vi "Aero_tunnel_monitor_on_OGI.vi"() -> ()   [LabVIEW 2015]
uses:
  Controls/Post_Process.ctl
  <vilib>/Platform/TimedLoop/XDataNode/timing_clust.ctl
  <vilib>/Platform/TimedLoop/XDataNode/nitl_modes.ctl
  <vilib>/Platform/TimedLoop/XDataNode/wakeup.ctl
  ADAM Client/Sub VIs/ADAM Controls/Update_scan_value.ctl
  <vilib>/Utility/file.llb/Write Delimited Spreadsheet (DBL).vi
  Globals/Meas_global.vi
  <vilib>/Platform/TimedLoop/XDataNode/XDataNode.xnode
  <vilib>/Platform/TimedLoop/XDataNode/XDNodeRunTimeDep.lvlib
panel:
  in  "Filename":path
  in  "Duration in Seconds":dbl=30.0
  in  "Log Full Res Balance data":bool
  in  "Use Polynomial for Ratio":bool
  in  "Manual Ratio":dbl=1.0075
  in  "Display Graph?":bool
  in  "Menu Ring":u16(ring) items=["Lift", "Pitch", "Drag", "Side", "Yaw", "Roll"]
  in  "Samples":i32=1000
  out "Waveform Chart":dbl[](graph)
  in  "Output Roll":bool
  out "Roll":string="0.0 Nm"
  in  "Output Yaw":bool
  out "Yaw":string="0.0 Nm"
  in  "Output Pitch":bool
  out "Pitch":string="0.0 Nm"
  in  "Output SF":bool
  out "SF":string="0.0 N"
  in  "Output Drag":bool
  out "Drag":string="0.0 N"
  in  "Output Lift":bool
  out "Lift":string="0.0 N"
  in  "Balance Safety limits":T1(array[cluster])=[{"Max +ve Range"=80, "Max -ve Range"=80, "Axis"="Lift"}, {"Max +ve Range"=80, "Max -ve Range"=80, "Axis"="Pitch"}, {"Max +ve Range"=80, "Max -ve Range"=80, "Axis"="Drag"}, {"Max +ve Range"=80, "Max -ve Range"=80, "Axis"="Side-Force"}, {"Max +ve Range"=99, "Max -ve Range"=99, "Axis"="Yaw"}, {"Max +ve Range"=80, "Max -ve Range"=80, "Axis"="Roll"}] {"Max -ve Range" min=0 max=125; "Max +ve Range" min=0 max=125}
  out "Monitor Speed (Hz)":dbl
  out "Belt slip warning":bool
  out "Road Status":string="???"
  in  "GotoYaw":bool
  in  "NewYawPos":dbl
  out "YAW POSITION":dbl
  out "Required WindSpeedRatio":dbl
  out "ROAD SPEED m/s":dbl
  in  "BL Fan1":i32
  in  "BL Fan2":i32
  in  "Stop drive":bool
  in  "Start Drive":bool
  in  "Synch to Wind":bool
  out "Road Info":string="???"
  in  "stop":bool
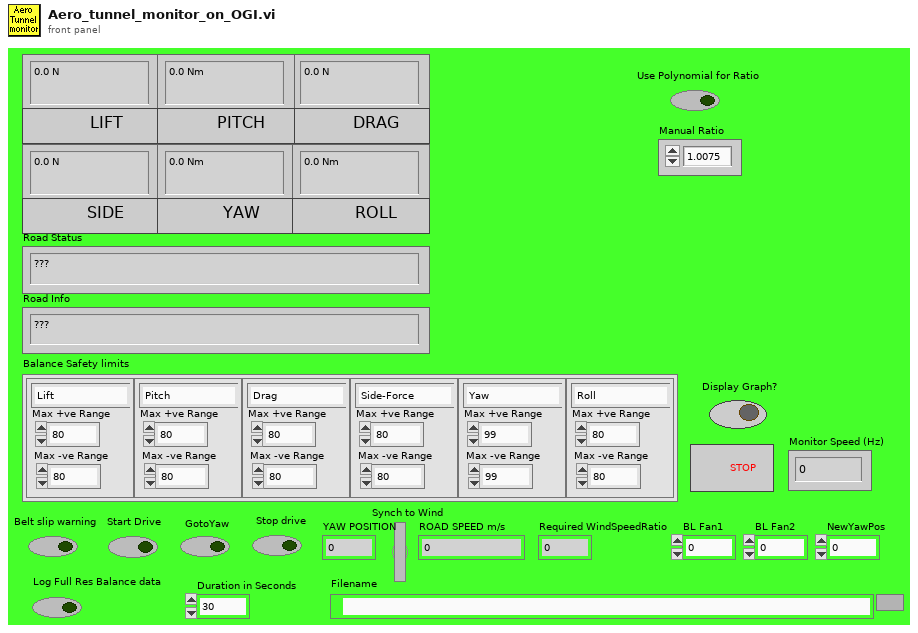
[diagram p1: front panel]
types:
  T1 = cluster{"Max +ve Range":i32, "Max -ve Range":i32, "Axis":string}[]
  T2 = typedef "Post_Process.ctl" = enum16{"Take New Data", "Post Process Raw Data File"}
  T3 = typedef "XDNodeRunTimeDep.lvlib/timing_clust.ctl" = cluster{"Expected End [f-1]":u64, "Actual End [f-1]":u64, "Finished Late? [f-1]":bool, "Expected End [i-1]":u64, "Actual End [i-1]":u64, "Finished Late? [i-1]":bool, "Expected Start [i]":u64, "Actual Start [i]":u64, "Expected Start [f]":u64, "Actual Start [f]":u64, "Source Name":string, "Structure Name":string, "Period":i64, "Deadline":i64, "Offset":i64, "Start":i64, "Priority":i32, "Timeout":i32, "Mode":T4, "Wakeup Reason":T5, "Error":errorcluster, "Source Type":string, "Secondary Source Type":string, "Global End Time":u64, "Global Start Time":u64, "Frame Duration":u64, "Iteration Duration":u64, "Assigned CPU":i32, "I/O Scan Engine Mode":u32}
  T4 = typedef "XDNodeRunTimeDep.lvlib/nitl_modes.ctl" = enum32{"No Change", "Process missed periods, maintain original phase", "Discard missed periods, maintain original phase", "Process missed periods, ignore original phase", "Discard missed periods, ignore original phase"}
  T5 = typedef "XDNodeRunTimeDep.lvlib/wakeup.ctl" = enum32{"Normal", "Aborted", "Asynchronous wakeup", "Timing source error", "Timed loop error", "Timeout"}
  T6 = typedef "Update_scan_value.ctl" = cluster{"Channel Name":string, "New Value":dbl}
  T7 = cluster{"Max +ve Range":i32, "Max -ve Range":i32, "Axis":string}
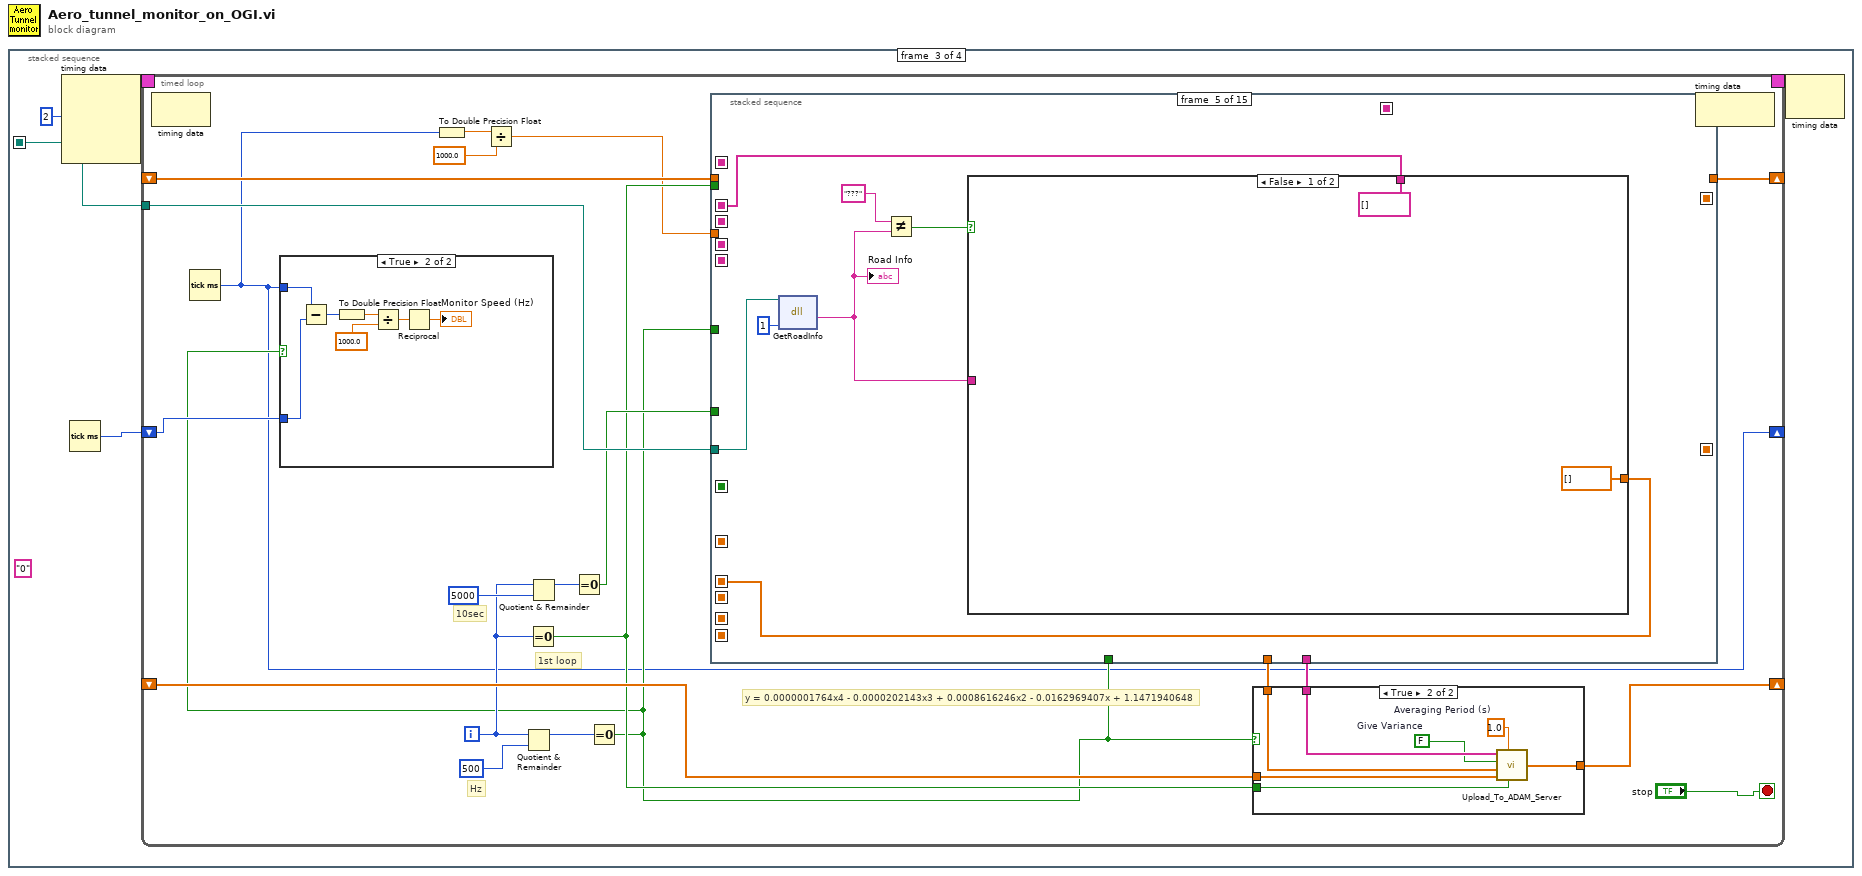
[diagram p0: block diagram]
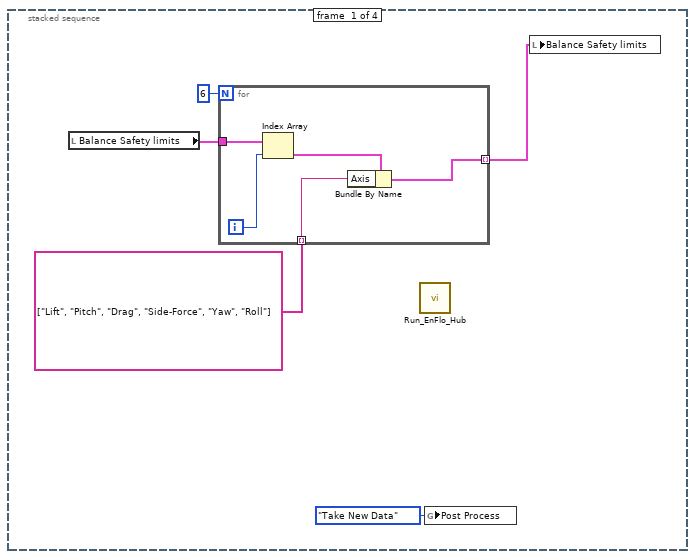
[diagram p2: hidden frame]
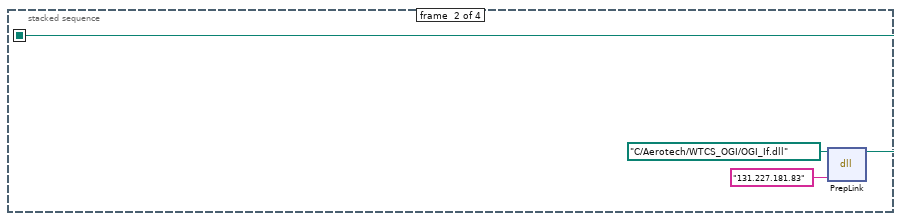
[diagram p3: hidden frame]
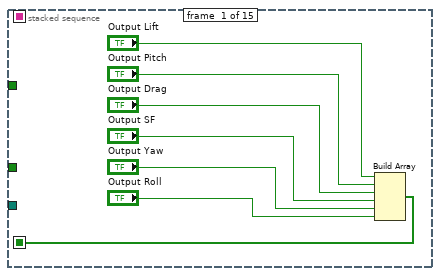
[diagram p6: hidden frame]
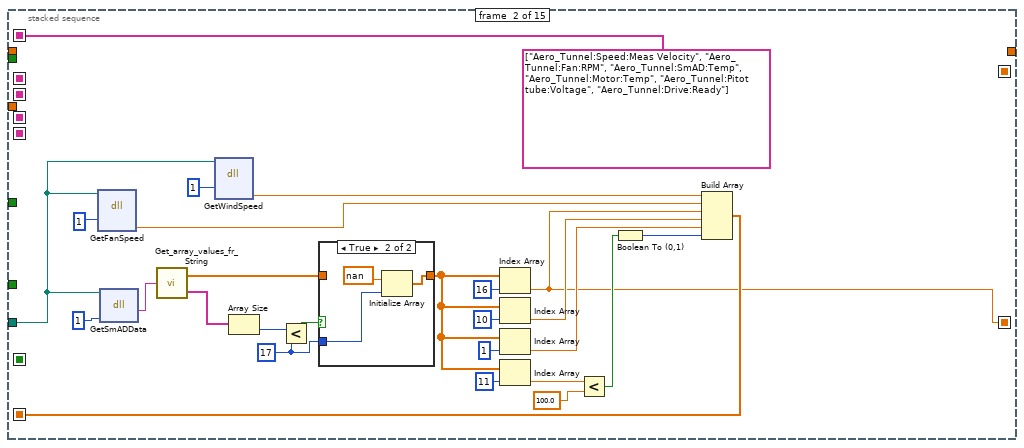
[diagram p7: hidden frame]
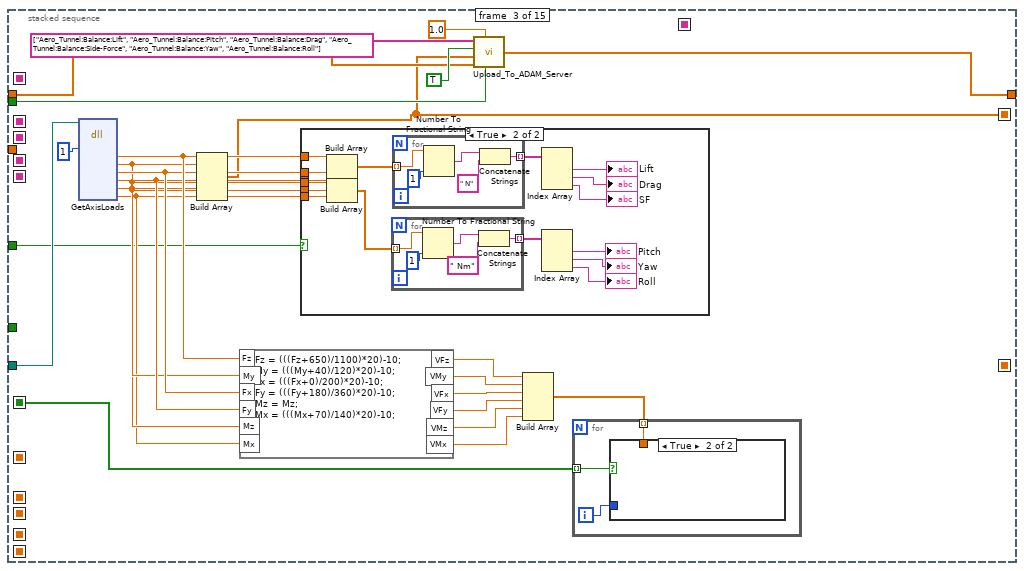
[diagram p9: hidden frame]
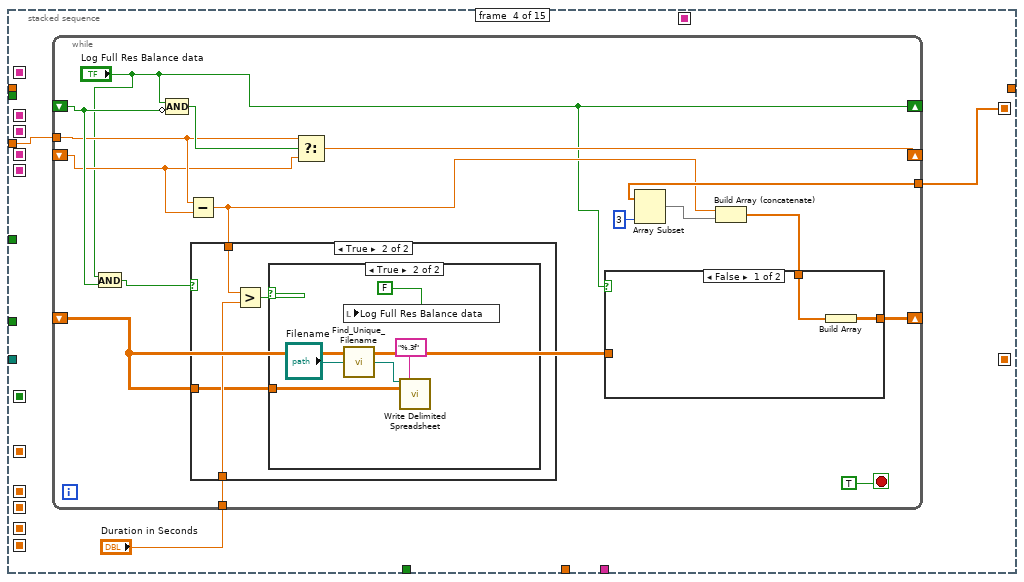
[diagram p12: hidden frame]
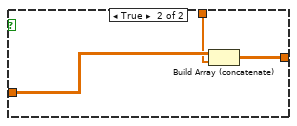
[diagram p13: hidden frame]
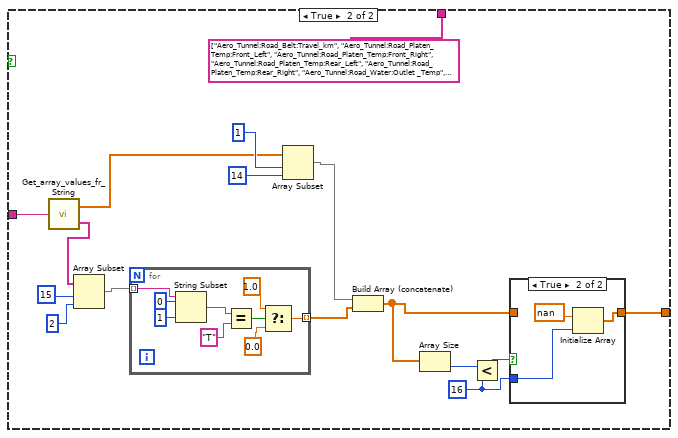
[diagram p16: hidden frame]
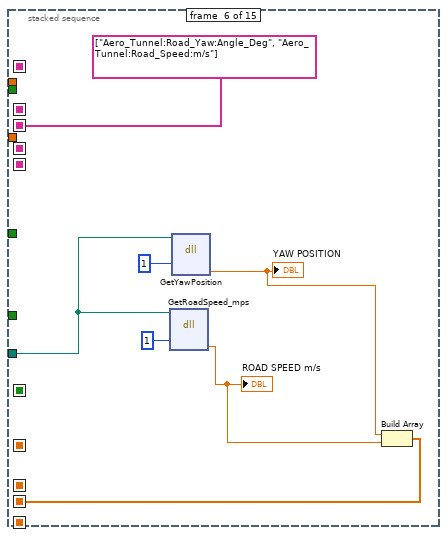
[diagram p18: hidden frame]
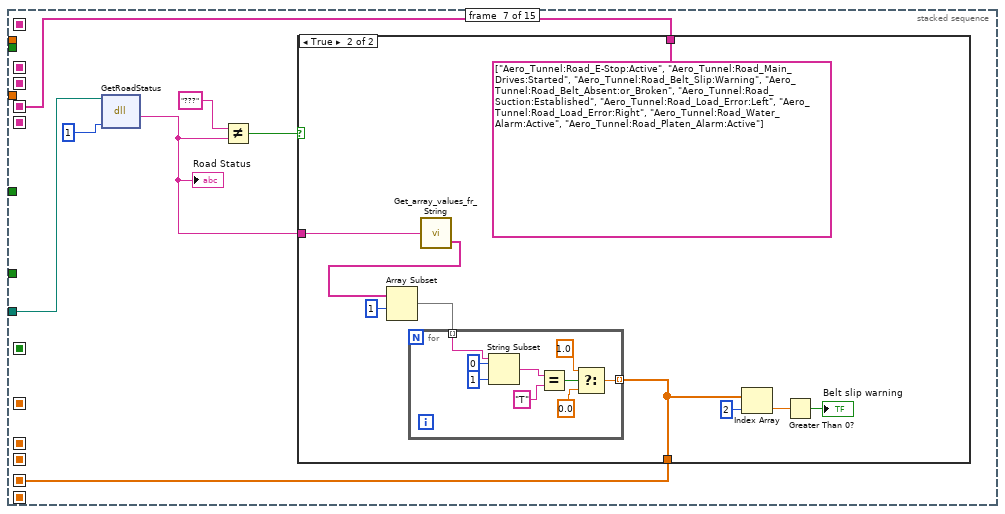
[diagram p19: hidden frame]
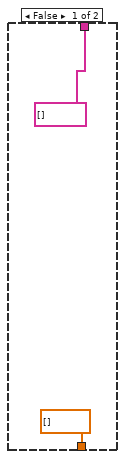
[diagram p20: hidden frame]
diagram:
  n1 = stacked-sequence {
    seq-local: [_ w11 _ _] -> [_ _ w18 w563]
    frame #0 {
      n2 = local read "Balance Safety limits"() -> (w4:T1)
      n3 = for {
        N: 6 -> [_]
        tunnel: w4 -> [w10]
        tunnel: [w7] -> w3 mode=indexing
        tunnel: string[] ["Lift", "Pitch", "Drag", "Side-Force", "Yaw", "Roll"] ("Channel Names") -> [w6] mode=indexing
        i -> [w9]
        n4 = Index Array(array=w10, index=w9) -> (element=w8:T7)
        n5 = Bundle By Name(cluster=w8, "Axis"=w6) -> (w7:T7)
      }
      n6 = call "Run_EnFlo_Hub.vi"() -> ()  [unwired: 8 in]
      n7 = global write "Meas_global.vi" "Post Process"(Post_Process."Take New Data" ("Post Process")) -> ()
      n8 = local write "Balance Safety limits"(w3) -> ()
    }
    frame #1 {
      n9 = dll-call lib="C:/Aerotech/Drivers/OGI_IF.dll" fn="PrepLink"(path in=path "C:/Aerotech/WTCS_OGI/OGI_If.dll", "IPAddress"="131.227.181.83") -> (path out=w11:path)  [unwired: 2 in, 3 out]
    }
    frame #2 {
      (unwired) "0" ("Channels")
      n10 = node-c288(i64 2 ("Period")) -> (w16:T3)  [unwired: 3 in]
      n11 = Tick Count (ms)() -> (millisecond timer value=w17:u32)
      n12 = timed-loop {
        shift-right: [w39] -> _
        shift-left: _ -> [w37]
        tunnel: w18 -> [w35]
        shift-right: [w33] -> _
        shift-left: _ -> [w34]
        timing: w16 -> [_]
        timing-out: [_] -> w15
        shift-right: [w22] -> _
        shift-left: w17 -> [w32]
        i -> [w26]
        stop <- "stop" stop-if-true
        # "1st loop"
        # "10sec"
        # "Hz"
        # "y = 0.0000001764x4 - 0.0000202143x3 + 0.0008616246x2 - 0.0162969407x + 1.1471940648"
        n13 = node-c288() -> ()  [unwired: 1 in, 1 out]
        n14 = Tick Count (ms)() -> (millisecond timer value=w22:u32)
        n15 = To Double Precision Float(number=w22) -> (double precision float=w20:dbl)
        n16 = Divide(x=w20, y=1000.0) -> (x/y=w19:dbl)
        n17 = Quotient & Remainder(x=w26, y=500) -> (x-y*floor(x/y)=w29:i32)  [unwired: 1 out]
        n18 = Equal To 0?(x=w26) -> (x = 0?=w25:bool)
        n19 = Quotient & Remainder(x=w26, y=5000) -> (x-y*floor(x/y)=w28:i32)  [unwired: 1 out]
        n20 = Equal To 0?(x=w28) -> (x = 0?=w27:bool)
        n21 = Equal To 0?(x=w29) -> (x = 0?=w24:bool)
        n22 = case shown="True" w24 {
          tunnel: w32 -> [_ w46]
          tunnel: w22 -> [_ w45]
          frame False {
          }
          frame True {
            n23 = Subtract(x=w45, y=w46) -> (x-y=w44:u32)
            n24 = To Double Precision Float(number=w44) -> (double precision float=w40:dbl)
            n25 = Divide(x=w40, y=1000.0) -> (x/y=w42:dbl)
            n26 = Reciprocal(x=w42) -> (1/x=→"Monitor Speed (Hz)":dbl)
          }
        }
        n27 = stacked-sequence {
          seq-local: [_ string[] ["Aero_Tunnel:Speed:Meas Velocity", "Aero_Tunnel:Fan:RPM", "Aero_Tunnel:SmAD:Temp", "Aero_Tunnel:Motor:Temp", "Aero_Tunnel:Pitot tube:Voltage", "Aero_Tunnel:Drive:Ready"] ("Channel Names") _ _ _ _ _ _ _ _ _ _ _ _ _] -> [_ _ _ _ _ _ _ _ _ _ _ w369 _ _ _]
          seq-local: [_ w79 _ _ _ _ _ _ _ _ _ _ _ _ _] -> [_ _ _ _ _ _ _ _ _ _ _ w368 _ _ _]
          seq-local: [_ _ _ _ w183 _ _ _ _ _ _ _ _ _ _] -> [_ _ _ _ _ _ _ _ _ _ _ w365 _ _ _]
          seq-local: [_ _ _ _ w184 _ _ _ _ _ _ _ _ _ _] -> [_ _ _ _ _ _ _ _ _ _ _ w354 _ _ _]
          seq-local: [_ _ _ _ _ string[] ["Aero_Tunnel:Road_Yaw:Angle_Deg", "Aero_Tunnel:Road_Speed:m/s"] ("Channel Names") _ _ _ _ _ _ _ _ _] -> [_ _ _ _ _ _ _ _ _ _ _ w364 _ _ _]
          seq-local: [_ _ _ _ _ w218 _ _ _ _ _ _ _ _ _] -> [_ _ _ _ _ _ _ _ _ _ _ w363 _ _ _]
          seq-local: [_ _ _ _ _ _ w229 _ _ _ _ _ _ _ _] -> [_ _ _ _ _ _ _ _ _ _ _ w359 _ _ _]
          seq-local: [_ _ _ _ _ _ w228 _ _ _ _ _ _ _ _] -> [_ _ _ _ _ _ _ _ _ _ _ w358 _ _ _]
          seq-local: [w57 _ _ _ _ _ _ _ _ _ _ _ _ _ _] -> [_ _ w109 _ _ _ _ _ _ _ _ _ _ _ _]
          seq-local: [_ _ _ _ _ _ _ string[] ["Aero_Tunnel:Balance_Range:Lift", "Aero_Tunnel:Balance_Range:Pitch", "Aero_Tunnel:Balance_Range:Drag", "Aero_Tunnel:Balance_Range:Side-Force", "Aero_Tunnel:Balance_Range:Yaw", "Aero_Tunnel:Balance_Range:Roll"] ("Channel Names") _ _ _ _ _ _ _] -> [_ _ _ _ _ _ _ _ _ _ _ w355 _ _ _]
          seq-local: [_ _ _ _ _ _ _ w253 _ _ _ _ _ _ _] -> [_ _ _ _ _ _ _ _ w284 _ _ w356 _ _ _]
          seq-local: [_ _ _ _ _ _ _ _ w280 _ _ _ _ _ _] -> [_ _ _ _ _ _ _ _ _ w314 w333 _ _ _ _]
          seq-local: [_ w64 _ _ _ _ _ _ _ _ _ _ _ _ _] -> [_ _ _ _ _ _ _ _ _ _ w332 _ _ _ _]
          seq-local: [_ _ w94 _ _ _ _ _ _ _ _ _ _ _ _] -> [_ _ _ w147 _ _ _ _ _ _ _ _ _ _ _]
          tunnel: [_ _ _ _ _ _ _ _ _ _ _ w367 _ _ _] -> w38
          tunnel: [_ _ _ _ _ _ _ _ _ _ _ w366 _ _ _] -> w36
          tunnel: w35 -> [_ w71 w116 _ w185 w221 w230 w262 _ _ _ w357 w371 w466 w493]
          tunnel: w24 -> [_ _ _ _ _ _ _ _ _ _ _ _ _ _ _]
          tunnel: w34 -> [_ _ w104 _ _ _ _ _ _ _ _ _ _ _ _]
          tunnel: [_ _ w103 _ _ _ _ _ _ _ _ _ _ _ _] -> w33
          tunnel: w24 -> [_ _ w96 _ _ _ _ _ _ _ _ _ w370 _ w492]
          tunnel: w27 -> [_ _ _ _ _ _ _ _ _ w313 _ _ _ w465 _]
          tunnel: w25 -> [_ _ w95 _ _ _ _ _ _ _ _ _ _ _ _]
          tunnel: w19 -> [_ _ _ w149 _ _ _ _ _ _ _ _ _ _ _]
          frame #0 {
            n28 = Build Array("Output Lift", "Output Pitch", "Output Drag", "Output SF", "Output Yaw", "Output Roll") -> (w57:bool[])
          }
          frame #1 {
            w65 = 17 ("y")
            n29 = dll-call lib="C:/Aerotech/Drivers/OGI_IF.dll" fn="GetFanSpeed"(path in=w71, "Enable"=1) -> ("FanSpeedinRPM"=w73:dbl)  [unwired: 3 in, 4 out]
            n30 = dll-call lib="C:/Aerotech/Drivers/OGI_IF.dll" fn="GetSmADData"(path in=w71, "Enable"=1) -> ("SmAD Data String"=w76:string)  [unwired: 2 in, 3 out]
            n31 = call "Get_array_values_fr_String.vi"("String Value"=w76) -> ("Numeric Array"=w66:dbl[], "String array"=w69:string[])
            n32 = dll-call lib="C:/Aerotech/Drivers/OGI_IF.dll" fn="GetWindSpeed"(path in=w71, "Enable"=1) -> ("Windspeed_M/s"=w72:dbl)  [unwired: 3 in, 4 out]
            n33 = Array Size(array=w69) -> (size(s)=w70:i32)
            n34 = Less?(x=w70, y=w65) -> (x < y?=w68:bool)
            n35 = case shown="True" w68 {
              tunnel: [w90 w93] -> w67
              tunnel: w66 -> [w90 _]
              tunnel: w65 -> [_ w91]
              frame False {
              }
              frame True {
                n36 = Initialize Array(nan, w91) -> (w93:dbl[])
              }
            }
            n37 = Index Array(array=w67, index=16) -> (element=w64:dbl)
            n38 = Index Array(array=w67, index=10) -> (element=w87:dbl)
            n39 = Index Array(array=w67, index=1) -> (element=w85:dbl)
            n40 = Index Array(array=w67, index=11) -> (element=w83:dbl)
            n41 = Less?(x=w83, y=100.0) -> (x < y?=w81:bool)
            n42 = Boolean To (0,1)(Boolean=w81) -> (0, 1=w80:i16)
            n43 = Build Array(w72, w73, w64, w87, w85, w80) -> (w79:dbl[])
          }
          frame #2 {
            n44 = dll-call lib="C:/Aerotech/Drivers/OGI_IF.dll" fn="GetAxisLoads"(path in=w116, "Enable"=1) -> ("Lift"=w102:dbl, "Pitch"=w99:dbl, "Drag"=w101:dbl, "side"=w100:dbl, "Yaw"=w98:dbl, "Roll"=w97:dbl)  [unwired: 3 in, 9 out]
            n45 = Build Array(w102, w99, w101, w100, w98, w97) -> (w94:dbl[])
            n46 = formula code="VFz = (((Fz+650)/1100)*20)-10;\nVMy = (((My+40)/120)*20)-10;\nVFx = (((Fx+0)/200)*20)-10;\nVFy = (((Fy+180)/360)*20)-10;\nVMz = Mz;\nVMx = (((Mx+70)/140)*20)-10;"("Fz"=w102, "My"=w99, "Fx"=w101, "Fy"=w100, "Mz"=w98, "Mx"=w97) -> ("VFz"=w115:dbl, "VMy"=w114:dbl, "VFx"=w113:dbl, "VFy"=w112:dbl, "VMz"=w111:dbl, "VMx"=w110:dbl)
            n47 = case shown="True" w96 {
              tunnel: w102 -> [_ w133]
              tunnel: w101 -> [_ w132]
              tunnel: w100 -> [_ w131]
              tunnel: w99 -> [_ w125]
              tunnel: w98 -> [_ w124]
              tunnel: w97 -> [_ w123]
              frame False {
              }
              frame True {
                n48 = Build Array(w133, w132, w131) -> (w130:dbl[])
                n49 = Build Array(w125, w124, w123) -> (w122:dbl[])
                n50 = for {
                  tunnel: w122 -> [w134] mode=indexing
                  tunnel: [w138] -> w121 mode=indexing
                  n51 = Number To Fractional String(number=w134, precision (6)=i16 1) -> (F-format string=w135:string)  [unwired: 2 in]
                  n52 = Concatenate Strings(w135, " Nm" ("string")) -> (w138:string)
                }
                n53 = for {
                  tunnel: w130 -> [w139] mode=indexing
                  tunnel: [w143] -> w129 mode=indexing
                  n54 = Number To Fractional String(number=w139, precision (6)=i16 1) -> (F-format string=w140:string)  [unwired: 2 in]
                  n55 = Concatenate Strings(w140, " N" ("string")) -> (w143:string)
                }
                n56 = Index Array(array=w129) -> (element #1=→"Lift":string, element #2=→"Drag":string, element #3=→"SF":string)  [unwired: 3 in]
                n57 = Index Array(array=w121) -> (element #1=→"Pitch":string, element #2=→"Yaw":string, element #3=→"Roll":string)  [unwired: 3 in]
              }
            }
            n58 = call "Upload_To_ADAM_Server.vi"("First Loop"=w95, "Averaging Period (s)"=1.0, "Shift In"=w104, "Channel Values"=w94, "Give Variance"=TRUE, "Channel Names"=string[] ["Aero_Tunnel:Balance:Lift", "Aero_Tunnel:Balance:Pitch", "Aero_Tunnel:Balance:Drag", "Aero_Tunnel:Balance:Side-Force", "Aero_Tunnel:Balance:Yaw", "Aero_Tunnel:Balance:Roll"]) -> ("Shift Out"=w103:dbl[])
            n59 = Build Array(w115, w114, w113, w112, w111, w110) -> (w108:dbl[])
            n60 = for {
              tunnel: w109 -> [w146] mode=indexing
              tunnel: w108 -> [w145] mode=indexing
              i -> [w144]
              n61 = case shown="True" w146 {
                tunnel: w145 -> [_ _]
                tunnel: w144 -> [_ _]
                frame False {
                }
                frame True {
                }
              }
            }
          }
          frame #3 {
            n62 = while {
              shift-right: ["Log Full Res Balance data"] -> _
              shift-left: _ -> [w163]
              shift-right: [w164] -> _
              shift-left: _ -> [w157]
              tunnel: w149 -> [w158]
              tunnel: "Duration in Seconds" -> [w161]
              tunnel: w147 -> [w159]
              shift-right: [w155] -> _
              shift-left: _ -> [w150]
              stop <- TRUE stop-if-true
              n63 = And(x="Log Full Res Balance data", y=w163) -> (x .and. y?=w162:bool)
              n64 = Compound Arithmetic op=AND("Log Full Res Balance data", invert w163) -> (w165:bool)
              n65 = Subtract(x=w158, y=w157) -> (x-y=w156:dbl)
              n66 = case shown="True" w162 {
                tunnel: w161 -> [_ w174]
                tunnel: w156 -> [_ w172]
                tunnel: w150 -> [_ w171]
                frame False {
                }
                frame True {
                  n67 = Greater?(x=w172, y=w174) -> (0:w173:bool)
                  n68 = case shown="True" w173 {
                    tunnel: w171 -> [_ w178]
                    frame False {
                    }
                    frame True {
                      n69 = local write "Log Full Res Balance data"(FALSE) -> ()
                      n70 = call "Find_Unique_Filename.vi"("Path In"="Filename") -> ("Unique Path Out"=w176:path)  [unwired: 2 in]
                      n71 = call-poly <vilib>:"Write Delimited Spreadsheet.vi"("file path (dialog if empty)"=w176, "format (%.3f)"="%.3f", "2D data"=w178) -> ()  [unwired: 11 in, 2 out]
                    }
                  }
                }
              }
              n72 = Select(t=w158, s=w165, f=w157) -> (s? t:f=w164:dbl)
              n73 = Array Subset(array=w159, length=3) -> (w153:dbl[])  [unwired: 1 in]
              n74 = Build Array (concatenate)(w156, w153) -> (w152:dbl[])
              n75 = case shown="False" "Log Full Res Balance data" {
                tunnel: [w166 w170] -> w155
                tunnel: w150 -> [_ w169]
                tunnel: w152 -> [w167 w168]
                frame False {
                  n76 = Build Array(w167) -> (w166:dbl[][])
                }
                frame True {
                  n77 = Build Array (concatenate)(w169, w168) -> (w170:dbl[][])
                }
              }
            }
          }
          frame #4 {
            n78 = dll-call lib="C:/Aerotech/Drivers/OGI_IF.dll" fn="GetRoadInfo"(path in=w185, "Enable"=1) -> ("Road Info"=w181:string)  [unwired: 3 in, 2 out]
            "Road Info" <- w181
            n79 = Not Equal?(x="???", y=w181) -> (x != y?=w180:bool)
            n80 = case shown="False" w180 {
              tunnel: [string[] [] ("Channel Names") string[] ["Aero_Tunnel:Road_Belt:Travel_km", "Aero_Tunnel:Road_Platen_Temp:Front_Left", "Aero_Tunnel:Road_Platen_Temp:Front_Right", "Aero_Tunnel:Road_Platen_Temp:Rear_Left", "Aero_Tunnel:Road_Platen_Temp:Rear_Right", "Aero_Tunnel:Road_Water:Outlet _Temp", "Aero_Tunnel:Road_Water:Inlet _Temp", "Aero_Tunnel:Road_Suction:Front", "Aero_Tunnel:Road_Suction:Middle", "Aero_Tunnel:Road_Suction:Rear", "Aero_Tunnel:Road_BL_Suction:Primary", "Aero_Tunnel:Road_BL_Suction:Secondary", "Aero_Tunnel:Road_LoadCell:Left", "Aero_Tunnel:Road_LoadCell:Right", "Aero_Tunnel:Road_Water_High:Temp_Alarm", "Aero_Tunnel:Road_Platen_High:Temp_Alarm"] ("Channel Names")] -> w184
              tunnel: [dbl[] [] w190] -> w183
              tunnel: w181 -> [_ w189]
              frame False {
              }
              frame True {
                w193 = 16 ("y")
                n81 = call "Get_array_values_fr_String.vi"("String Value"=w189) -> ("Numeric Array"=w192:dbl[], "String array"=w196:string[])
                n82 = Array Subset(array=w196, index=15, length=2) -> (w200:string[])
                n83 = for {
                  tunnel: w200 -> [w215] mode=indexing
                  tunnel: [w209] -> w199 mode=indexing
                  n84 = String Subset(string=w215, offset (0)=0, length (rest)=1 ("length (rest)")) -> (substring=w214:string)
                  n85 = Equal?(x=w214, y="T") -> (x = y?=w212:bool)
                  n86 = Select(t=1.0, s=w212, f=0.0) -> (s? t:f=w209:dbl)
                }
                n87 = Array Subset(array=w192, index=1, length=14) -> (w198:dbl[])
                n88 = Build Array (concatenate)(w198, w199) -> (w191:dbl[])
                n89 = Array Size(array=w191) -> (size(s)=w195:i32)
                n90 = Less?(x=w195, y=w193) -> (x < y?=w194:bool)
                n91 = case shown="True" w194 {
                  tunnel: [w205 w208] -> w190
                  tunnel: w191 -> [w205 _]
                  tunnel: w193 -> [_ w206]
                  frame False {
                  }
                  frame True {
                    n92 = Initialize Array(nan, w206) -> (w208:dbl[])
                  }
                }
              }
            }
          }
          frame #5 {
            n93 = dll-call lib="C:/Aerotech/Drivers/OGI_IF.dll" fn="GetRoadSpeed_mps"(path in=w221, "Enable"=1) -> ("RoadSpeed_mps"=w219:dbl)  [unwired: 3 in, 4 out]
            "ROAD SPEED m/s" <- w219
            n94 = dll-call lib="C:/Aerotech/Drivers/OGI_IF.dll" fn="GetYawPosition"(path in=w221, "Enable"=1) -> ("Yaw Position"=w220:dbl)  [unwired: 3 in, 4 out]
            "YAW POSITION" <- w220
            n95 = Build Array(w220, w219) -> (w218:dbl[])
          }
          frame #6 {
            n96 = dll-call lib="C:/Aerotech/Drivers/OGI_IF.dll" fn="GetRoadStatus"(path in=w230, "Enable"=1) -> ("Road Status"=w227:string)  [unwired: 3 in, 2 out]
            "Road Status" <- w227
            n97 = Not Equal?(x="???", y=w227) -> (x != y?=w225:bool)
            n98 = case shown="True" w225 {
              tunnel: [string[] [] ("Channel Names") string[] ["Aero_Tunnel:Road_E-Stop:Active", "Aero_Tunnel:Road_Main_Drives:Started", "Aero_Tunnel:Road_Belt_Slip:Warning", "Aero_Tunnel:Road_Belt_Absent:or_Broken", "Aero_Tunnel:Road_Suction:Established", "Aero_Tunnel:Road_Load_Error:Left", "Aero_Tunnel:Road_Load_Error:Right", "Aero_Tunnel:Road_Water_Alarm:Active", "Aero_Tunnel:Road_Platen_Alarm:Active"] ("Channel Names")] -> w229
              tunnel: [dbl[] [] w241] -> w228
              tunnel: w227 -> [_ w234]
              frame False {
              }
              frame True {
                n99 = call "Get_array_values_fr_String.vi"("String Value"=w234) -> ("String array"=w237:string[])  [unwired: 1 out]
                n100 = Array Subset(array=w237, index=1) -> (w235:string[])  [unwired: 1 in]
                n101 = for {
                  tunnel: [w244] -> w241 mode=indexing
                  tunnel: w235 -> [w243] mode=indexing
                  n102 = String Subset(string=w243, offset (0)=0, length (rest)=1 ("length (rest)")) -> (substring=w249:string)
                  n103 = Equal?(x=w249, y="T") -> (x = y?=w247:bool)
                  n104 = Select(t=1.0, s=w247, f=0.0) -> (s? t:f=w244:dbl)
                }
                n105 = Index Array(array=w241, index=2) -> (element=w239:dbl)
                n106 = Greater Than 0?(x=w239) -> (x > 0?=→"Belt slip warning":bool)
              }
            }
          }
          frame #7 {
            n107 = dll-call lib="C:/Aerotech/Drivers/OGI_IF.dll" fn="GetAxisPercs"(path in=w262, "Enable"=1) -> ("Lift"=w260:dbl, "Pitch"=w259:dbl, "Drag"=w258:dbl, "side"=w257:dbl, "Yaw"=w256:dbl, "Roll"=w255:dbl)  [unwired: 3 in, 9 out]
            n108 = Build Array(w260, w259, w258, w257, w256, w255) -> (w253:dbl[])
            n109 = case shown="True" "Display Graph?" {
              selector: "Display Graph?" -> [w263 w264]
              tunnel: w253 -> [_ w268]
              frame False {
                n110 = property on="Waveform Chart" class="WFChart (strict)"("Visible"=w263) -> ()  [unwired: 2 in, 2 out]
                n111 = property on="Samples" class="DigNum (strict)"("Visible"=w263) -> ()  [unwired: 2 in, 2 out]
                n112 = property on="Menu Ring" class="Ring (strict)"("Visible"=w263) -> ()  [unwired: 2 in, 2 out]
              }
              frame True {
                n113 = while {
                  shift-right: [w270] -> _
                  shift-left: _ -> [w272]
                  tunnel: w268 -> [w271]
                  tunnel: [w270] -> w267
                  stop <- TRUE stop-if-true
                  n114 = for {
                    tunnel: w272 -> [w275]
                    tunnel: w271 -> [w273] mode=indexing
                    tunnel: [w278] -> w270 mode=indexing
                    i -> [w276]
                    n115 = Index Array(array=w275, index (row)=w276) -> (element=w274:dbl[])  [unwired: 1 in]
                    n116 = Build Array (concatenate)(w273, w274) -> (w279:dbl[])
                    n117 = Array Subset(array=w279, length="Samples") -> (w278:dbl[])  [unwired: 1 in]
                  }
                }
                n118 = Index Array(array=w267, index (row)="Menu Ring") -> (element=→"Waveform Chart":dbl[])  [unwired: 1 in]
                n119 = property on="Waveform Chart" class="WFChart (strict)"("Visible"=w264) -> ()  [unwired: 2 in, 2 out]
                n120 = property on="Samples" class="DigNum (strict)"("Visible"=w264) -> ()  [unwired: 2 in, 2 out]
                n121 = property on="Menu Ring" class="Ring (strict)"("Visible"=w264) -> ()  [unwired: 2 in, 2 out]
              }
            }
          }
          frame #8 {
            n122 = for {
              tunnel: "Balance Safety limits" -> [w300] mode=indexing
              tunnel: w284 -> [w303] mode=indexing
              shift-right: [w297] -> w281
              shift-left: "" -> [w298]
              n123 = To Long Integer(number=w303) -> (32bit integer=w299:i32)
              n124 = Unbundle By Name(w300) -> ("Max +ve Range"=w305:i32, "Max -ve Range"=w304:i32)
              n125 = Negate(x=w304) -> (-x=w302:i32)
              n126 = In Range and Coerce(upper limit=w305, x=w299, lower limit=w302) -> (In Range?=w301:bool)  [unwired: 1 out]
              n127 = case shown="False" w301 {
                tunnel: w300 -> [w311 _]
                tunnel: w299 -> [w309 _]
                tunnel: w298 -> [w307 w312]
                tunnel: [w306 w312] -> w297
                frame False {
                  n128 = Unbundle By Name(w311) -> ("Axis"=w310:string)
                  n129 = Format Into String(format string="The %s is at %d%% of its range.\n", initial string=w307, w310, w309) -> (resulting string=w306:string)  [unwired: 1 in, 1 out]
                }
                frame True {
                }
              }
            }
            n130 = Empty String/Path?(string/path=w281) -> (empty?=w282:bool)
            n131 = case shown="False" w282 {
              tunnel: w281 -> [w288 w296]
              tunnel: [w286 w296] -> w280
              frame False {
                n132 = Build Array("Aero_Tunnel:Fan:Watchdog") -> (w295:string[])
                n133 = call "Get_Current_Scan_client.vi"("ADAM Ch Names"=w295) -> ("Numerical Values"=w293:dbl[])  [unwired: 1 in, 2 out]
                n134 = Index Array(array=w293, index=0) -> (element=w291:dbl)
                n135 = Greater?(x=w291, y=0.5) -> (0:w289:bool)
                n136 = Select(t=w288, s=w289, f="") -> (s? t:f=w286:string)
              }
              frame True {
              }
            }
          }
          frame #9 {
            n137 = while {
              tunnel: w314 -> [w318]
              tunnel: w313 -> [w315]
              stop <- TRUE stop-if-true
              n138 = Empty String/Path?(string/path=w318) -> (empty?=w320:bool)
              n139 = Not(x=w320) -> (.not. x?=w316:bool)
              n140 = Compound Arithmetic op=AND(w316, w315) -> (w319:bool)
              n141 = case shown="True" w319 {
                tunnel: w318 -> [_ w325]
                frame False {
                }
                frame True {
                  w324 = string[] ["Aero_Tunnel:Fan:Watchdog", "Aero_Tunnel:Road:Watchdog", "Aero_Tunnel:Speed:Dem Velocity"] ("Channel Names")
                  n142 = Format Into String(format string="The Aero Tunnel balance has gone outside of its limits.\n%s\nThe Aero_Tunnel:Fan:Watchdog has therefore been disabled. ", w325) -> (resulting string=w326:string)  [unwired: 2 in, 1 out]
                  n143 = Bundle By Name(cluster=errorcluster {"status"=TRUE, "code"=0, "source"=""} ("error in (no error)"), "source"=w326) -> (w328:errorcluster)
                  n144 = Array Size(array=w324) -> (size(s)=w323:i32)
                  n145 = call "EnFlo_Error_Handler.vi"("error in (no error)"=w328, "Error Type"="Aero Tunnel Balance Range Trip", "Dialog Box (T)"=FALSE) -> ()  [unwired: 3 out]
                  n146 = Initialize Array(0.0, w323) -> (w321:dbl[])
                  n147 = call "ASYNC_Adam_client.vi"("Values"=w321, "Channel Names"=w324) -> ()  [unwired: 1 in, 2 out]
                }
              }
            }
          }
          frame #10 {
            n148 = while {
              tunnel: w333 -> [_]
              shift-right: [w338] -> _
              shift-left: _ -> [w337]
              tunnel: w332 -> [w335]
              stop <- TRUE stop-if-true
              n149 = Greater?(x=w335, y=35.0) -> (0:w338:bool)
              n150 = Number To Fractional String(number=w335, precision (6)=i16 2) -> (F-format string=w334:string)  [unwired: 2 in]
              n151 = Compound Arithmetic op=AND(invert w337, w338) -> (w341:bool)
              n152 = case shown="True" w341 {
                tunnel: w334 -> [_ w346]
                frame False {
                }
                frame True {
                  w345 = string[] ["Aero_Tunnel:Fan:Watchdog", "Aero_Tunnel:Road:Watchdog", "Aero_Tunnel:Speed:Dem Velocity"] ("Channel Names")
                  n153 = Format Into String(format string="The Aero Tunnel temperature has gone above it's limits and is:\n%s\nThe Aero_Tunnel:Fan:Watchdog has therefore been disabled. ", w346) -> (resulting string=w347:string)  [unwired: 2 in, 1 out]
                  n154 = Bundle By Name(cluster=errorcluster {"status"=TRUE, "code"=0, "source"=""} ("error in (no error)"), "source"=w347) -> (w349:errorcluster)
                  n155 = Array Size(array=w345) -> (size(s)=w344:i32)
                  n156 = call "EnFlo_Error_Handler.vi"("error in (no error)"=w349, "Error Type"="Aero Tunnel Temperature Trip", "Dialog Box (T)"=FALSE) -> ()  [unwired: 3 out]
                  n157 = Initialize Array(0.0, w344) -> (w342:dbl[])
                  n158 = call "ASYNC_Adam_client.vi"("Values"=w342, "Channel Names"=w345) -> ()  [unwired: 1 in, 2 out]
                }
              }
            }
          }
          frame #11 {
            n159 = Build Array (concatenate)(w368, w365, w363, w358, w356) -> (w367:dbl[])
            n160 = Boolean To (0,1)(Boolean="GotoYaw") -> (0, 1=w362:i16)
            n161 = Build Array (concatenate)(w369, w354, w364, w359, w355) -> (w366:string[])
            n162 = To Long Integer(number=w362) -> (32bit integer=w353:i32)
            n163 = dll-call lib="C:/Aerotech/Drivers/OGI_IF.dll" fn="GotoYawPosition"(path in=w357, "Enable"=w353, "NewYawPos"="NewYawPos") -> ()  [unwired: 3 in, 4 out]
          }
          frame #12 {
            n164 = case shown="True" w370 {
              tunnel: w371 -> [_ w372]
              frame False {
              }
              frame True {
                # "Tweak"
                # "Speed"
                # "Tweak"
                # "Speed"
                n165 = stacked-sequence {
                  seq-local: [_ w386 _ _ _ _] -> [_ _ _ w431 _ _]
                  seq-local: [_ w377 _ _ _ _] -> [_ _ _ w427 _ _]
                  seq-local: [_ w384 _ _ _ _] -> [_ _ _ _ w447 _]
                  seq-local: [_ w380 _ _ _ _] -> [_ _ _ _ _ w456]
                  seq-local: [_ w378 _ _ _ _] -> [_ _ _ _ _ _]
                  seq-local: [_ w376 _ _ _ _] -> [_ _ _ _ _ _]
                  seq-local: [string[] ["Aero_Tunnel:Speed:Dem Velocity", "Froude:NPL:Atmos_Press", "Aero_Tunnel:Motor:Enable", "Aero_Tunnel:Speed:Calib Tweak", "Aero_Tunnel:Upper:Temp", "Aero_Tunnel:Lower:Temp", "Aero_Tunnel:Fan:Watchdog"] ("appended array") _ _ _ _ _] -> [_ w375 _ _ _ _]
                  seq-local: [_ w374 _ _ _ _] -> [_ _ w410 _ _ _]
                  tunnel: w372 -> [_ w388 _ w430 w446 w457]
                  frame #0 {
                  }
                  frame #1 {
                    n166 = call "Get_Current_Scan_client.vi"("ADAM Ch Names"=w375) -> ("Numerical Values"=w374:dbl[])  [unwired: 1 in, 2 out]
                    n167 = Index Array(array=w374, index=0) -> (element=w386:dbl)
                    n168 = Index Array(array=w374, index=3) -> (element=w378:dbl)
                    n169 = Index Array(array=w374, index=1) -> (element=w384:dbl)
                    n170 = while {
                      tunnel: w388 -> [w396]
                      tunnel: w386 -> [w395]
                      shift-right: [w395] -> _
                      shift-left: _ -> [w394]
                      shift-right: [w391] -> _
                      shift-left: _ -> [w392]
                      tunnel: w378 -> [w391]
                      tunnel: [w390] -> w377
                      tunnel: [w389] -> w376
                      stop <- TRUE stop-if-true
                      n171 = Not Equal?(x=w395, y=w394) -> (x != y?=w390:bool)
                      n172 = Not Equal?(x=w391, y=w392) -> (x != y?=w389:bool)
                      n173 = case shown="True" w390 {
                        tunnel: w396 -> [_ w397]
                        tunnel: w395 -> [_ w398]
                        frame False {
                        }
                        frame True {
                          n174 = Greater?(x=w398, y=0.2) -> (0:w399:bool)
                          n175 = Boolean To (0,1)(Boolean=w399) -> (0, 1=w402:i16)
                          n176 = dll-call lib="C:/Aerotech/Drivers/OGI_IF.dll" fn="SetFanSystemState"(path in=w397, "Enable"=1, "Fan ONOFF"=w402) -> ()  [unwired: 3 in, 4 out]
                        }
                      }
                    }
                    n177 = Index Array(array=w374, index=2) -> (element=w382:dbl)
                    n178 = Greater?(x=w382, y=0.5) -> (0:w380:bool)
                  }
                  frame #2 {
                    # "allowed temp."
                    n179 = Index Array(array=w410, index=6) -> (element=w408:dbl)
                    n180 = Array Subset(array=w410, index=4, length=3) -> (w412:dbl[])
                    n181 = Array Max & Min(array=w412) -> (max value=w403:dbl)  [unwired: 3 out]
                    n182 = Greater?(x=w408, y=0.5) -> (0:w405:bool)
                    n183 = Greater?(x=w403, y=35.0) -> (0:w406:bool)
                    n184 = And(x=w406, y=w405) -> (x .and. y?=w404:bool)
                    n185 = case shown="True" w404 {
                      tunnel: w403 -> [_ w417]
                      frame False {
                      }
                      frame True {
                        n186 = Format Into String(format string="Aero Tunnel temp is %.1f. The Aero_Tunnel:Fan:Watchdog has therefore been disabled. ", w417) -> (resulting string=w415:string)  [unwired: 2 in, 1 out]
                        n187 = Bundle By Name(cluster=errorcluster {"status"=TRUE, "code"=0, "source"=""} ("error in (no error)"), "source"=w415) -> (w418:errorcluster)
                        n188 = call "EnFlo_Error_Handler.vi"("error in (no error)"=w418, "Error Type"="Aero Tunnel over temp", "Dialog Box (T)"=FALSE) -> ()  [unwired: 3 out]
                        n189 = call "ASYNC_Adam_client.vi"("Values"=dbl[] [0.0, 0.0], "Channel Names"=string[] ["Aero_Tunnel:Fan:Watchdog", "Aero_Tunnel:Road:Watchdog"]) -> ()  [unwired: 1 in, 2 out]
                      }
                    }
                  }
                  frame #3 {
                    n190 = feedback-in #1("Manual Ratio") -> ()
                    n191 = feedback #1() -> (w429:dbl)  [unwired: 1 in]
                    n192 = Not Equal?(x="Manual Ratio", y=w429) -> (x != y?=w425:bool)
                    n193 = Or(x=w425, y=w427) -> (x .or. y?=w426:bool)
                    n194 = case shown="True" w426 {
                      tunnel: w431 -> [_ w439]
                      tunnel: w430 -> [_ w445]
                      tunnel: "Manual Ratio" -> [_ w433]
                      tunnel: "Use Polynomial for Ratio" -> [_ w435]
                      frame False {
                      }
                      frame True {
                        (unwired) dbl[] [0.7807, 0.0283, -0.0013, 2e-05] ("Calib constants")
                        # "no fillets no rolling road no suction"
                        # "rolling road full suction fillets"
                        n195 = call "Polynomial_convert.vi"("Calib constants"=dbl[] [1.1471940648, -0.0162969407, 0.0008616246, -2.02143e-05, 1.764e-07], "Voltage"=w439) -> ("Eng Values"=w434:dbl)  [unwired: 4 in]
                        n196 = Select(t=w434, s=w435, f=w433) -> (s? t:f=w432:dbl)
                        n197 = Equal To 0?(x=w439) -> (x = 0?=w440:bool)
                        n198 = In Range and Coerce(upper limit=1.12, x=w432, lower limit=0.88) -> (coerced(x)=w437:dbl)  [unwired: 1 out]
                        n199 = Select(t=0.88, s=w440, f=w437) -> (s? t:f=w436:dbl)
                        "Required WindSpeedRatio" <- w436
                        n200 = dll-call lib="C:/Aerotech/Drivers/OGI_IF.dll" fn="SetWindSpeedRatio"(path in=w445, "Enable"=1 ("t"), "Required WindSpeedRatio"=w436) -> ()  [unwired: 4 in, 3 out]
                      }
                    }
                  }
                  frame #4 {
                    n201 = while {
                      shift-right: [w449] -> _
                      shift-left: _ -> [w452]
                      tunnel: w447 -> [w449]
                      tunnel: w446 -> [w450]
                      stop <- TRUE stop-if-true
                      n202 = Equal?(x=w449, y=w452) -> (x = y?=w451:bool)
                      n203 = case shown="True" w451 {
                        tunnel: w450 -> [_ w455]
                        tunnel: w449 -> [_ w453]
                        frame False {
                        }
                        frame True {
                          n204 = dll-call lib="C:/Aerotech/Drivers/OGI_IF.dll" fn="SetNewbaroPr_mB"(path in=w455, "Enable"=1, "NewPressure"=w453) -> ()  [unwired: 3 in, 4 out]
                        }
                      }
                    }
                  }
                  frame #5 {
                    n205 = while {
                      shift-right: [w460] -> _
                      shift-left: _ -> [w459]
                      tunnel: w456 -> [w460]
                      tunnel: w457 -> [w462]
                      stop <- TRUE stop-if-true
                      n206 = Compound Arithmetic op=AND(w460, invert w459) -> (w458:bool)
                      n207 = case shown="True" w458 {
                        tunnel: w462 -> [_ w464]
                        frame False {
                        }
                        frame True {
                          n208 = dll-call lib="C:/Aerotech/Drivers/OGI_IF.dll" fn="SetPitotZero"(path in=w464, "Enable"=1) -> ()  [unwired: 2 in, 4 out]
                        }
                      }
                    }
                  }
                }
              }
            }
          }
          frame #13 {
            n209 = while {
              tunnel: w466 -> [w473]
              shift-right: [w471] -> _
              shift-left: _ -> [w470]
              tunnel: w465 -> [w469]
              shift-right: [w467] -> _
              shift-left: _ -> [w468]
              stop <- TRUE stop-if-true
              # "Do every 10 seconds"
              n210 = case shown="True" w469 {
                tunnel: w473 -> [_ _]
                tunnel: [w475 w489] -> w471
                tunnel: w470 -> [w475 w488]
                tunnel: w468 -> [w474 w480]
                tunnel: [w474 w478] -> w467
                frame False {
                  (unwired) FALSE
                }
                frame True {
                  # "Do every 10 minutes"
                  # "flip flop every 10 cycles"
                  n211 = Increment(x=w480) -> (x+1=w477:i32)
                  n212 = Greater?(x=w477, y=60) -> (0:w476:bool)
                  n213 = case shown="False" w476 {
                    tunnel: [w490 0] -> w478
                    tunnel: w477 -> [w490 _]
                    frame False {
                    }
                    frame True {
                    }
                  }
                  n214 = Select(t=1.0, s=w488, f=0.0) -> (s? t:f=w482:dbl)
                  n215 = Bundle By Name(cluster=T6 {"Channel Name"="Aero_Tunnel:Server:Pulse", "New Value"=0.0} ("Update Scan Value Cluster"), "New Value"=w482) -> (w484:T6)
                  n216 = Not(x=w488) -> (.not. x?=w489:bool)
                  n217 = Build Array(w484) -> (w483:T6[])
                  n218 = call "Update_Current_Value_client.vi"("Don't Bother with check?"=TRUE, "Update array in"=w483) -> ()
                }
              }
            }
          }
          frame #14 {
            n219 = while {
              shift-right: [w504] -> _
              shift-left: _ -> [w506]
              tunnel: w492 -> [w505]
              tunnel: w493 -> [w502]
              shift-right: [w500] -> _
              shift-left: _ -> [w501]
              shift-right: [w498] -> _
              shift-left: _ -> [w499]
              shift-right: [w495] -> _
              shift-left: _ -> [w497]
              shift-right: [w494] -> _
              shift-left: _ -> [w496]
              stop <- TRUE stop-if-true
              n220 = stacked-sequence {
                tunnel: w506 -> [w512 _ _ _]
                tunnel: w505 -> [w510 w528 w538 w550]
                tunnel: ["Synch to Wind" _ _ _] -> w504
                tunnel: w502 -> [w507 w526 w536 w552]
                tunnel: w501 -> [_ w525 _ _]
                tunnel: [_ "Start Drive" _ _] -> w500
                tunnel: w499 -> [_ _ w535 _]
                tunnel: [_ _ "Stop drive" _] -> w498
                tunnel: w497 -> [_ _ _ w549]
                tunnel: w496 -> [_ _ _ w546]
                tunnel: [_ _ _ "BL Fan1"] -> w495
                tunnel: [_ _ _ "BL Fan2"] -> w494
                frame #0 {
                  n221 = Not Equal?(x="Synch to Wind", y=w512) -> (x != y?=w511:bool)
                  n222 = Or(x=w511, y=w510) -> (x .or. y?=w508:bool)
                  n223 = case shown="False" w508 {
                    tunnel: "Synch to Wind" -> [_ w521]
                    tunnel: w507 -> [w513 w520]
                    frame False {
                      n224 = Build Array("Aero_Tunnel:Road:Dem_Velocity") -> (w517:string[])
                      n225 = call "Get_Current_Scan_client.vi"("ADAM Ch Names"=w517) -> ("Numerical Values"=w516:dbl[])  [unwired: 1 in, 2 out]
                      n226 = Index Array(array=w516) -> (element=w515:dbl)  [unwired: 1 in]
                      n227 = dll-call lib="C:/Aerotech/Drivers/OGI_IF.dll" fn="SetRoadSpeed_mps"(path in=w513, "Enable"=1, "Required_mps"=w515) -> ()  [unwired: 3 in, 4 out]
                    }
                    frame True {
                      n228 = Boolean To (0,1)(Boolean=w521) -> (0, 1=w522:i16)
                      n229 = To Long Integer(number=w522) -> (32bit integer=w519:i32)
                      n230 = dll-call lib="C:/Aerotech/Drivers/OGI_IF.dll" fn="RoadSyncToWind"(path in=w520, "Enable"=1, "SynchState"=w519) -> ()  [unwired: 3 in, 4 out]
                    }
                  }
                }
                frame #1 {
                  n231 = Not Equal?(x="Start Drive", y=w525) -> (x != y?=w529:bool)
                  n232 = Or(x=w529, y=w528) -> (x .or. y?=w527:bool)
                  n233 = case shown="True" w527 {
                    tunnel: "Start Drive" -> [_ w533]
                    tunnel: w526 -> [_ w531]
                    frame False {
                    }
                    frame True {
                      n234 = Boolean To (0,1)(Boolean=w533) -> (0, 1=w532:i16)
                      n235 = To Long Integer(number=w532) -> (32bit integer=w530:i32)
                      n236 = dll-call lib="C:/Aerotech/Drivers/OGI_IF.dll" fn="StartRoadDrive"(path in=w531, "Enable"=w530) -> ()  [unwired: 2 in, 4 out]
                    }
                  }
                }
                frame #2 {
                  n237 = Not Equal?(x="Stop drive", y=w535) -> (x != y?=w539:bool)
                  n238 = Or(x=w539, y=w538) -> (x .or. y?=w537:bool)
                  n239 = case shown="True" w537 {
                    tunnel: "Stop drive" -> [_ w543]
                    tunnel: w536 -> [_ w541]
                    frame False {
                    }
                    frame True {
                      n240 = Boolean To (0,1)(Boolean=w543) -> (0, 1=w542:i16)
                      n241 = To Long Integer(number=w542) -> (32bit integer=w540:i32)
                      n242 = dll-call lib="C:/Aerotech/Drivers/OGI_IF.dll" fn="RoadStop"(path in=w541, "Enable"=w540) -> ()  [unwired: 2 in, 4 out]
                    }
                  }
                }
                frame #3 {
                  n243 = Not Equal?(x=w546, y="BL Fan2") -> (x != y?=w547:bool)
                  n244 = Not Equal?(x="BL Fan1", y=w549) -> (x != y?=w548:bool)
                  n245 = Compound Arithmetic op=OR(w548, w547, w550) -> (w551:bool)
                  n246 = case shown="True" w551 {
                    tunnel: w552 -> [_ w554]
                    tunnel: "BL Fan1" -> [_ w556]
                    tunnel: "BL Fan2" -> [_ w555]
                    frame False {
                    }
                    frame True {
                      w553 = 1 ("BL Fan (1 or 2)")
                      n247 = dll-call lib="C:/Aerotech/Drivers/OGI_IF.dll" fn="SetBoundaryPerc"(path in=w554, "enable"=w553, "BL Fan (1 or 2)"=1, "New Percentage"=w556) -> ()  [unwired: 4 in, 4 out]
                      n248 = dll-call lib="C:/Aerotech/Drivers/OGI_IF.dll" fn="SetBoundaryPerc"(path in=w554, "enable"=w553, "BL Fan (1 or 2)"=2, "New Percentage"=w555) -> ()  [unwired: 4 in, 4 out]
                    }
                  }
                }
              }
            }
          }
        }
        n249 = case shown="True" w24 {
          tunnel: [w49 w56] -> w39
          tunnel: w38 -> [_ w55]
          tunnel: w37 -> [w49 w54]
          tunnel: w36 -> [_ w53]
          tunnel: w25 -> [_ w50]
          frame False {
          }
          frame True {
            w51 = FALSE  # Give Variance
            w52 = 1.0  # Averaging Period (s)
            n250 = call "Upload_To_ADAM_Server.vi"("First Loop"=w50, "Averaging Period (s)"=w52, "Shift In"=w54, "Channel Values"=w55, "Give Variance"=w51, "Channel Names"=w53) -> ("Shift Out"=w56:dbl[])
          }
        }
        n251 = node-c288() -> ()  [unwired: 1 in, 1 out]
      }
      n252 = node-c288(w15) -> ()  [unwired: 1 out]
    }
    frame #3 {
      n253 = dll-call lib="C:/Aerotech/Drivers/OGI_IF.dll" fn="CloseLink"(path in=w563) -> ()  [unwired: 2 in, 3 out]
    }
  }
